vi "Radius Check.vi"(11 "Component In":T1) -> (3 "R in range?":bool)   [LabVIEW 2021, in "Component Tray.lvclass"]
uses:
  Component Tray.lvclass
  Find Component.ctl
  Controller/Camera/Machine Vision.ctl
  Component Tray.lvclass/Component Tray.ctl
  Controller/Camera/Camera.lvclass
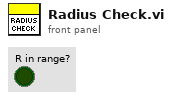
[diagram p1: front panel]
types:
  T1 = typedef "Component Tray.lvclass/Find Component.ctl" = cluster{"New Fiducials":dbl[], "Past Fiducials":dbl[][], "XYZTheta":dbl[], "Fiducials Path":path, "Position":i32, "CH1 Location":dbl[], "Sensor ID Location":dbl[], "initial rotation":dbl[], "CH2 location":dbl[], "max std variation":dbl, "max strength":dbl, "CH2 pattern matching":T2, "Fiducial Circle":T2, "Get Edge":T2, "Pos multiplier":dbl, "time to wait":u32, "fiducial to edge":dbl, "Protomodule?":bool, "Assembly Type":string, "CH1 to CH2":dbl, "Tray Number":string, "fiducial radius":dbl, "4 fiducials?":bool, "CH1 check":T2, "Edge Scan":T2, "CH1 pattern matching":T2, "Sensor Thickness":dbl}
  T2 = typedef "Camera.lvclass/Machine Vision.ctl" = enum16{"None", "Assembly Tray Circle", "Assembly Tray Fiducial", "Partial Hexaboard", "sensor edge init", "HB edge init", "sensor edge pos1", "sensor edge pos2", "HB edge pos1", "HB edge pos2", "Sensor CH1-2", "HB CH1", "HB CH2", "V3 Sensor Circle", "Hexaboard Circle", "sensor CH1 check", "HB CH1 check "}
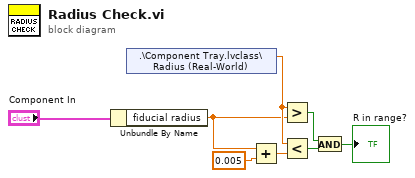
[diagram p0: block diagram]
diagram:
  n1 = Unbundle By Name("Component In") -> ("fiducial radius"=w3:dbl)
  n2 = shared-variable ".\\Component Tray.lvclass\\Radius (Real-World)"() -> (w7:dbl)  [unwired: 1 in, 1 out]
  n3 = Add(x=w3, y=0.005) -> (x+y=w6:dbl)
  n4 = Greater?(x=w7, y=w3) -> (0:w2:bool)
  n5 = Less?(x=w7, y=w6) -> (x < y?=w8:bool)
  n6 = And(x=w2, y=w8) -> (x .and. y?=→"R in range?":bool)
